vi "controlPanel.vi"() -> ()   [LabVIEW 2019]
panel:
  out "Error Out":errorcluster
  out "SetYPosition":dbl
  out "SetXPosition":dbl
  out "Equation":string
  out "NormalVector":dbl[](array[numeric])
  out "D":dbl
  out "Three Points":dbl[][](array[numeric])
  in  "Sim/live":bool
  out "Position":dbl[](array[numeric])
  in  "Zaxis Step Size":dbl
  out "SytemID":i32
  out "AxisID":string[](array[string])
  out "Ready":bool
  in  "stop":bool
  # "A"
  # "B"
  # "C"
  # "X"
  # "Y"
  # "Z"
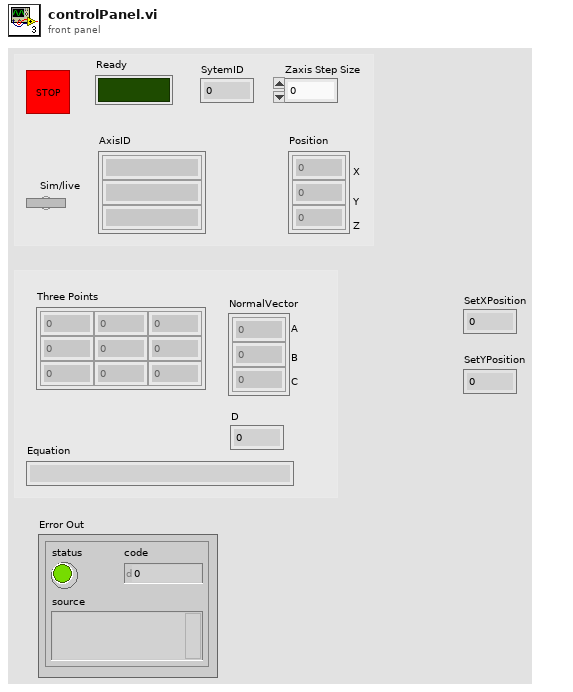
[diagram p1: front panel]
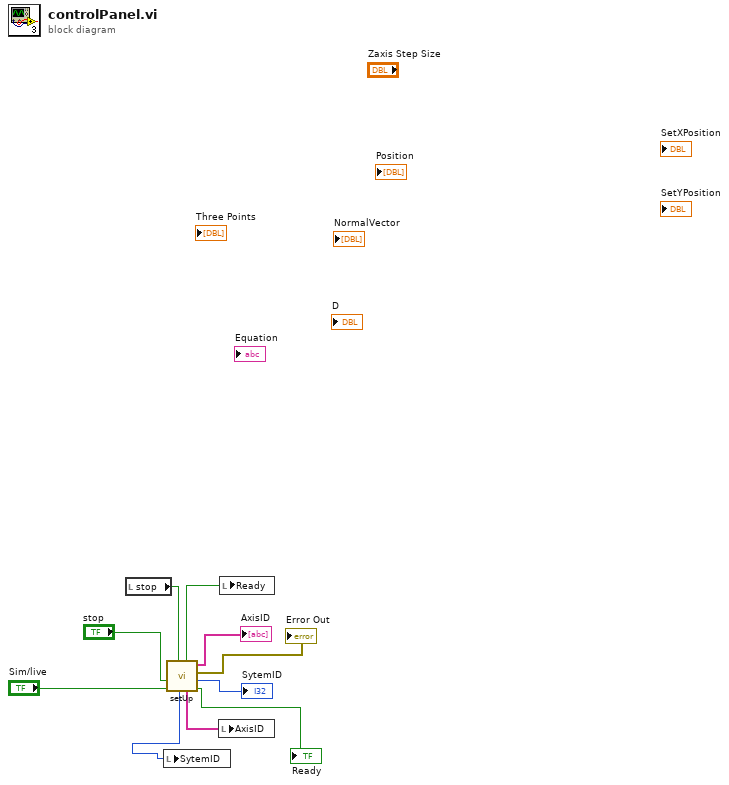
[diagram p0: block diagram]
diagram:
  n1 = local read "stop"() -> (w5:bool)
  n2 = call "setUp.vi"("stop 2"=w5, "live/Sim"="Sim/live", "stop"="stop") -> ("Ready"=→"Ready":bool, "SystemID"=→"SytemID":i32, "Error Out"=→"Error Out":errorcluster, "AxisID"=→"AxisID":string[], "AxisID 2"=w8:string[], "Ready 2"=w3:bool, "SystemID 2"=w1:i32)  [unwired: 2 in]
  n3 = local write "SytemID"(w1) -> ()
  n4 = local write "AxisID"(w8) -> ()
  n5 = local write "Ready"(w3) -> ()
